vi "Injection Test.vi"(10 "Progress":string, 11 "ProgressText":string) -> (3 "EndTestText":string)   [LabVIEW 2012]
panel:
  in  "milliseconds to wait":u32=10000
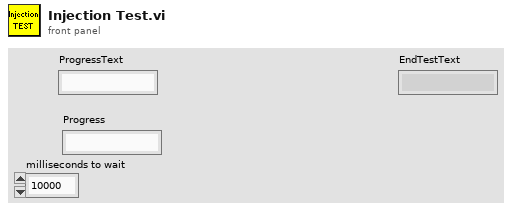
[diagram p1: front panel]
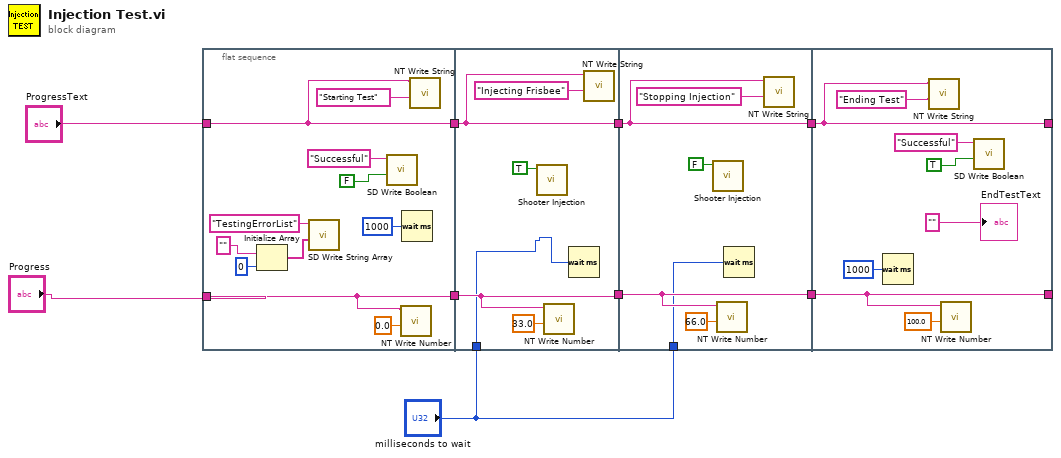
[diagram p0: block diagram]
diagram:
  n1 = flat-sequence {
    tunnel: "ProgressText" -> [w16]
    tunnel: "Progress" -> [w19]
    tunnel: [w16] -> w9
    tunnel: [w19] -> w8
    tunnel: w9 -> [w24]
    tunnel: w8 -> [w26]
    tunnel: [w24] -> w7
    tunnel: [w26] -> w6
    tunnel: "milliseconds to wait" -> [w21]
    tunnel: w7 -> [w29]
    tunnel: w6 -> [w28]
    tunnel: [w29] -> w3
    tunnel: [w28] -> w2
    tunnel: "milliseconds to wait" -> [w27]
    tunnel: [w33] -> _
    tunnel: [w34] -> _
    tunnel: w3 -> [w34]
    tunnel: w2 -> [w33]
    frame #0 {
      n2 = Initialize Array("", 0 ("dimension size")) -> (w11:string[])
      n3 = call <vilib>:"SD Write String Array.vi"("String Array"=w11, "Name"="TestingErrorList") -> ()  [unwired: 8 in, 2 out]
      n4 = call <vilib>:"SD Write Boolean.vi"("Boolean"=FALSE, "Name"="Successful") -> ()  [unwired: 8 in, 2 out]
      n5 = call <vilib>:"NT Write Number.vi"("Numeric"=0.0, "Name"=w19) -> ()  [unwired: 9 in, 1 out]
      n6 = Wait (ms)(milliseconds to wait=u32 1000) -> ()  [unwired: 1 out]
      n7 = call <vilib>:"NT Write String.vi"("String"="Starting Test", "Name"=w16) -> ()  [unwired: 9 in, 1 out]
    }
    frame #1 {
      n8 = call "Shooter Injection.vi"("Inject"=TRUE) -> ()  [unwired: 11 in]
      n9 = call <vilib>:"NT Write Number.vi"("Numeric"=33.0, "Name"=w26) -> ()  [unwired: 9 in, 1 out]
      n10 = Wait (ms)(milliseconds to wait=w21) -> ()  [unwired: 1 out]
      n11 = call <vilib>:"NT Write String.vi"("String"="Injecting Frisbee", "Name"=w24) -> ()  [unwired: 9 in, 1 out]
    }
    frame #2 {
      n12 = call "Shooter Injection.vi"("Inject"=FALSE) -> ()  [unwired: 11 in]
      n13 = call <vilib>:"NT Write Number.vi"("Numeric"=66.0, "Name"=w28) -> ()  [unwired: 9 in, 1 out]
      n14 = Wait (ms)(milliseconds to wait=w27) -> ()  [unwired: 1 out]
      n15 = call <vilib>:"NT Write String.vi"("String"="Stopping Injection", "Name"=w29) -> ()  [unwired: 9 in, 1 out]
    }
    frame #3 {
      n16 = Wait (ms)(milliseconds to wait=u32 1000) -> ()  [unwired: 1 out]
      n17 = call <vilib>:"NT Write String.vi"("String"="Ending Test", "Name"=w34) -> ()  [unwired: 9 in, 1 out]
      n18 = call <vilib>:"NT Write Number.vi"("Numeric"=100.0, "Name"=w33) -> ()  [unwired: 9 in, 1 out]
      n19 = call <vilib>:"SD Write Boolean.vi"("Boolean"=TRUE, "Name"="Successful") -> ()  [unwired: 8 in, 2 out]
      "EndTestText" <- "" ("EndTestText")
    }
  }
